vi "Wczytaj_wartosci_z_INI.vi"(7 "Section":string, 8 "error in (no error)":errorcluster, 10 "key names":string[](array[string]), 11 "refnum":T1) -> (0 "error out":errorcluster, 2 "Array":dbl[](array[numeric]), 3 "refnum out":T1)   [LabVIEW 2014]
doc: "Wczytuje wszystkie klucze (boolean) z zadanej sekcji"
uses:
  <vilib>/Utility/config.llb/Config Data RefNum.ctl
  <vilib>/Utility/config.llb/Read Key (Double).vi
  <vilib>/Utility/config.llb/NI_LVConfig.lvlib
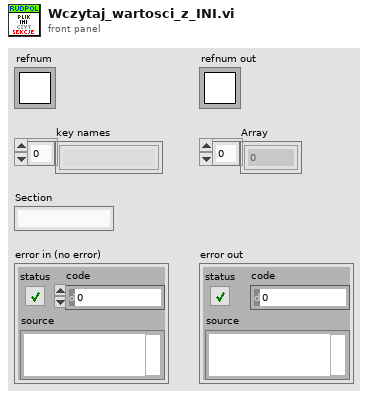
[diagram p1: front panel]
types:
  T1 = typedef "NI_LVConfig.lvlib/Config Data RefNum.ctl" = refnum<k1>
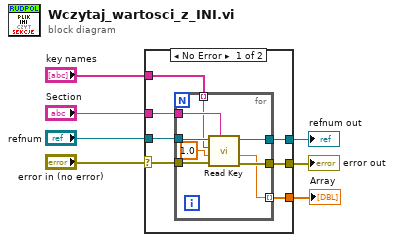
[diagram p0: block diagram]
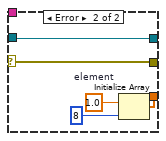
[diagram p2: hidden frame]
diagram:
  n1 = case shown="No Error" "error in (no error)" {
    selector: "error in (no error)" -> [w8 w27]
    tunnel: [w14 w26] -> w7
    tunnel: [w13 w27] -> w6
    tunnel: [w12 w25] -> w5
    tunnel: "Section" -> [w11 _]
    tunnel: "key names" -> [w10 _]
    tunnel: "refnum" -> [w9 w26]
    frame No Error {
      n2 = for {
        tunnel: w8 -> [w22]
        tunnel: w9 -> [w21]
        tunnel: w10 -> [w19] mode=indexing
        tunnel: w11 -> [w20]
        tunnel: [w17] -> w14
        tunnel: [w16] -> w13
        tunnel: [w15] -> w12 mode=indexing
        n3 = call-poly <vilib>:"Read Key.vi"("section"=w20, "error in (no error)"=w22, "default value"=1.0, "key"=w19, "refnum"=w21) -> ("error out"=w16:errorcluster, "value"=w15:dbl, "refnum out"=w17:T1)  [unwired: 3 in, 1 out]
      }
    }
    frame Error {
      w24 = 1.0  # element
      n4 = Initialize Array(w24, 8) -> (w25:dbl[])
    }
  }
  "refnum out" <- w7
  "error out" <- w6
  "Array" <- w5
